vi "initialize.vi"(0 "HGF_TaskEventListener":refnum<class "HGF_TaskEventListener.lvclass">, 3 "initializationData":variant, 5 "error in (no error)":errorcluster, 7 "binaryString":string, 8 "I8 Array":i8[](array[numeric]), 9 "prependSize? (T)":bool, 11 "byteOrder (0:big-endian, network order)":T1(ring)) -> (14 "dup HGF_TaskEventListener":refnum<class "HGF_TaskEventListener.lvclass">, 17 "found?":bool, 19 "error out":errorcluster)   [LabVIEW 2012, in "HGF_ObjectManager.lvlib" / "HGF_TaskEventListener.lvclass"]
doc: "This is a dynamic dispatch VI to be implemented by child classes to initialize their attributes.\n\n<B>Recommendation:</B> Use Variant for initialization data."
uses:
  HGF_TaskEventListener.lvclass
  HGF_ThreadTask/HGF_ThreadTask.lvclass
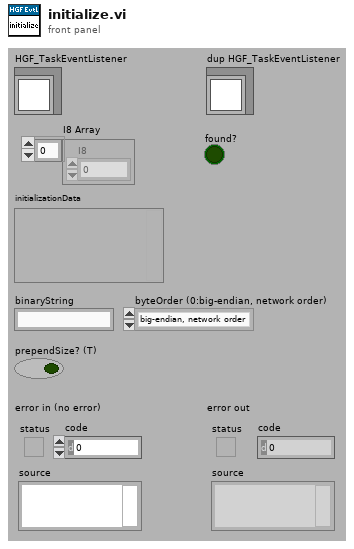
[diagram p1: front panel]
types:
  T1 = enum16{"big-endian, network order", "native, host order", "little-endian"}
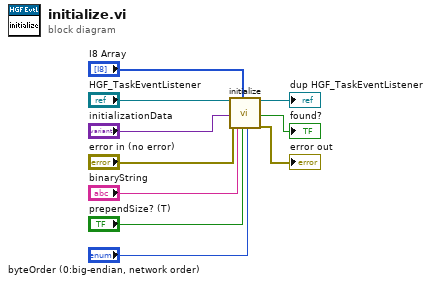
[diagram p0: block diagram]
diagram:
  n1 = call-parent "initialize.vi"("HGF_ThreadTask"="HGF_TaskEventListener", "initializationData"="initializationData", "error in (no error)"="error in (no error)", "binaryString"="binaryString", "I8 Array"="I8 Array", "prependSize? (T)"="prependSize? (T)", "byteOrder (0:big-endian, network order)"="byteOrder (0:big-endian, network order)") -> ("dup HGF_ThreadTask"=→"dup HGF_TaskEventListener":refnum<class "HGF_TaskEventListener.lvclass">, "found?"=→"found?":bool, "error out"=→"error out":errorcluster)  [unwired: 10 out]
